vi "Temp2700RunFix.vi"(8 "error in":errorcluster, 10 "Fix Mode":bool, 11 "VISA resource name":refnum<visa-resource-name>) -> (0 "error out":errorcluster, 2 "Success":bool, 3 "VISA resource name out":refnum<visa-resource-name>)   [LabVIEW 2016]
doc: "Activate FIX operation Run"
uses:
  <instrlib>/Samwontech TEMP2xxx/Samwontech TEMP2xxx.lvlib
panel:
  out "Response (original)":string
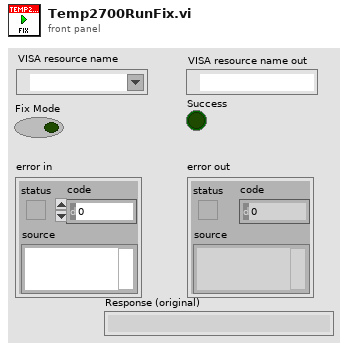
[diagram p1: front panel]
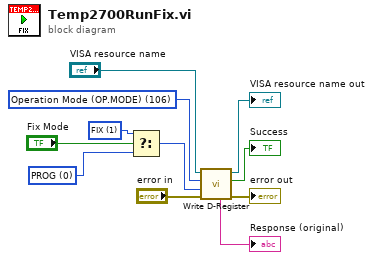
[diagram p0: block diagram]
diagram:
  w7 = u32 0 items=["PROG", "FIX"] ("Operation Mode")
  w8 = u32 1 items=["PROG", "FIX"] ("Operation Mode")
  w10 = u32 106 items=["Current PV (NPV)"=1, "Operation Control (COM.OPMODE)"=102, "Set Point on FIX operation (FIX.TSP)"=104, "Operation Mode (OP.MODE)"=106] ("D-Registers Map")
  n1 = Select(t=w8, s="Fix Mode", f=w7) -> (s? t:f=w1:u32)
  n2 = call <instrlib>:"Write D-Register.vi"("error in"="error in", "Data"=w1, "D-register number"=w10, "VISA resource name"="VISA resource name") -> ("error out"=→"error out":errorcluster, "Successfully"=→"Success":bool, "VISA resource name out"=→"VISA resource name out":refnum<visa-resource-name>, "Responce (original)"=→"Response (original)":string)  [unwired: 4 in]
